vi "Engine Library Name.vi"() -> (3 "Engine Library Name":string)   [LabVIEW 2019, in "DSF Core.lvlib" / "Framework.lvclass"]
uses:
  Classes/Framework/Framework.lvclass
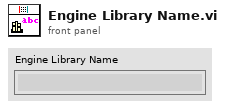
[diagram p1: front panel]
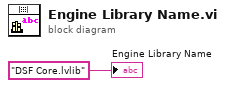
[diagram p0: block diagram]
diagram:
  "Engine Library Name" <- "DSF Core.lvlib" ("Library Name")
